vi "Test Stubs.vi"   [LabVIEW 2014]
uses:
  Controller/Controller.lvclass
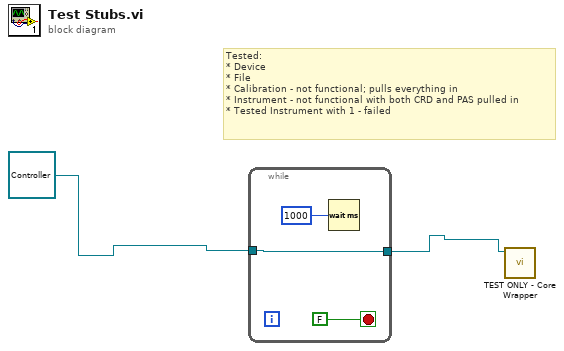
[diagram p0: block diagram]
diagram:
  # "Tested:\n* Device\n* File\n* Calibration - not functional; pulls everything in\n* Instrument - not functional with both CRD and PAS pulled in\n* Tested Instrument with 1 - failed"
  n1 = while {
    tunnel: refnum<class "Controller.lvclass"> refnum ("Controller:Controller") -> [w4]
    tunnel: [w4] -> w2
    stop <- FALSE stop-if-true
    n2 = Wait (ms)(milliseconds to wait=u32 1000) -> ()  [unwired: 1 out]
  }
  n3 = call-dynamic "TEST ONLY - Core Wrapper.vi"("Ex Nested in"=w2) -> ()  [unwired: 10 in, 1 out]
